vi "LF Read File (STR)__ogtk.vi"(4 "type":string, 5 "convert eol (F)":bool, 6 "bytes to read":i32, 7 "line mode (F)":bool, 8 "error in (no error)":errorcluster, 9 "offset in (0)":dbl, 10 "pos mode (current)":enum16{"start", "end", "current"}(ring)=enum."current", 11 "refnum":refnum<file>) -> (0 "error out":errorcluster, 1 "offset out":dbl, 2 "String":string, 3 "refnum out":refnum<file>)   [LabVIEW 2018]
doc: "Reads a string using a double precision number as offset to work for files larger than 2GB."
uses:
  kernel32.dll
panel:
  # "not implemented"
  # "max offset is limited to about\n2^51 (1 000 000 000 000 000)  bytes\nto maintain full resolution of 1 bytes"
  # "LF Read File (STR).vi\n\nPlease visit http://www.OpenG.org to learn about the\nOpen Source LabVIEW software movement.\n\nNOTICE -- YOU MUST LEAVE THIS NOTICE IN PLACE.  PER THE TERMS OF THE LICENSE BELOW, YOU MAY SUBLICENSE THIS SOFTWARE \nIN ANY WAY THAT DOES NOT CONFLICT WITH THIS LICENSE.\n\n### BSD License (http://www.opensource.org/licenses/bsd-license.php) Begin ###\n\nCopyright (c) 2003, Rolf Kalbermatter <rolf.kalbermatter@citeng.com>\n\nAll rights reserved.\n\nRedistribution and use in source and binary forms, with or without modification, are permitted provided that the following conditions are met:\n\n    * Redistributions of source code must retain the above copyright notice, this list of conditions and the following disclaimer.\n    * Redistributions in binary form must reproduce the above copyright notice, this list of conditions and the following disclaimer in the \n       documentation and/or other materials provided with the distribution.\n    * Neither the name of SciWare, James Kring, Inc., nor the names of its contributors may be used to endorse or promote products derived \n       from this software without specific prior written permission.\n\nTHIS SOFTWARE IS PROVIDED BY THE COPYRIGHT HOLDERS AND CONTRIBUTORS \"AS IS\" AND ANY EXPRESS OR IMPLIED WARRANTIES, \nINCLUDING, BUT NOT LIMITED TO, THE IMPLIED WARRANTIES OF MERCHANTABILITY AND FITNESS FOR A PARTICULAR PURPOSE ARE \nDISCLAIMED. IN NO EVENT SHALL THE COPYRIGHT OWNER OR CONTRIBUTORS BE LIABLE FOR ANY DIRECT, INDIRECT, INCIDENTAL,\n SPECIAL, EXEMPLARY, OR CONSEQUENTIAL DAMAGES (INCLUDING, BUT NOT LIMITED TO, PROCUREMENT OF SUBSTITUTE GOODS OR \nSERVICES; LOSS OF USE, DATA, OR PROFITS; OR BUSINESS INTERRUPTION) HOWEVER CAUSED AND ON ANY THEORY OF LIABILITY, \nWHETHER IN CONTRACT, STRICT LIABILITY, OR TORT (INCLUDING NEGLIGENCE OR OTHERWISE) ARISING IN ANY WAY OUT OF THE USE \nOF THIS SOFTWARE, EVEN IF ADVISED OF THE POSSIBILITY OF SUCH DAMAGE.\n\n### BSD License End ###"
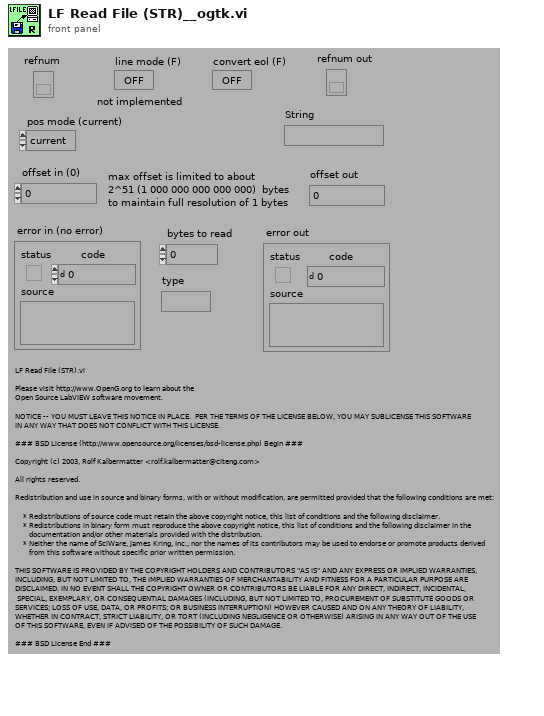
[diagram p1: front panel]
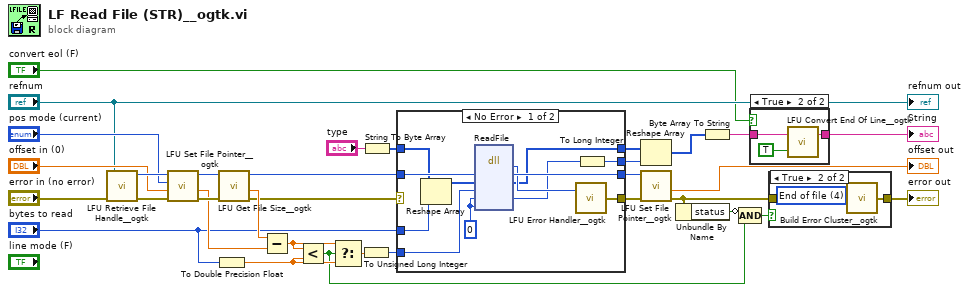
[diagram p0: block diagram]
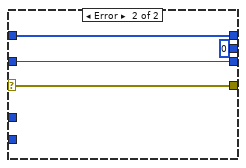
[diagram p4: hidden frame]
diagram:
  n1 = call <userlib>:"LFU Retrieve File Handle__ogtk.vi"("error in (no error)"="error in (no error)", "file refnum"="refnum") -> ("error out"=w31:errorcluster, "handle out"=w32:u32)  [unwired: 4 in]
  n2 = call <userlib>:"LFU Set File Pointer__ogtk.vi"("error in (no error)"=w31, "offset in (0)"="offset in (0)", "pos mode (current)"="pos mode (current)", "handle"=w32) -> ("error out"=w27:errorcluster, "offset out"=w24:dbl, "handle out"=w26:u32)  [unwired: 1 in]
  n3 = To Double Precision Float(number="bytes to read") -> (double precision float=w22:dbl)
  n4 = call <userlib>:"LFU Get File Size__ogtk.vi"("error in (no error)"=w27, "handle"=w26) -> ("error out"=w16:errorcluster, "file size"=w23:dbl, "handle out"=w13:u32)  [unwired: 3 in]
  n5 = Subtract(x=w23, y=w24) -> (x-y=w21:dbl)
  n6 = Less?(x=w21, y=w22) -> (x < y?=w18:bool)
  n7 = Select(t=w21, s=w18, f=w22) -> (s? t:f=w20:dbl)
  n8 = To Unsigned Long Integer(number=w20) -> (unsigned 32bit integer=w14:u32)
  n9 = String To Byte Array(string="type") -> (unsigned byte array=w12:u8[])
  n10 = case shown="No Error" w16 {
    selector: w16 -> [_ w48]
    tunnel: [w45 w49] -> w8
    tunnel: w13 -> [w44 w49]
    tunnel: [w43 w48] -> w4
    tunnel: w14 -> [w41 _]
    tunnel: w12 -> [w39 w47]
    tunnel: "bytes to read" -> [w38 _]
    tunnel: [w36 w47] -> w10
    tunnel: [w35 0 ("bytesRead")] -> w9
    frame No Error {
      w37 = u32 0 ("overlapped")
      n11 = Reshape Array(w39, w38) -> (w40:u8[])
      n12 = dll-call lib="kernel32.dll" fn="ReadFile"("handle"=w44, "buffer"=w40, "bytesToRead"=w41, "bytesRead"=w37, "overlapped"=w37) -> (w42:u32, "handle"=w45:u32, "buffer"=w36:u8[], "bytesRead"=w34:u32)  [unwired: 5 in, 2 out]
      n13 = call <userlib>:"LFU Error Handler__ogtk.vi"("retval"=w42) -> ("error out"=w43:errorcluster)  [unwired: 1 in]
      n14 = To Long Integer(number=w34) -> (32bit integer=w35:i32)
    }
    frame Error {
      (unwired) u32 0 ("bytesRead")
    }
  }
  n15 = Reshape Array(w10, w9) -> (w7:u8[])
  n16 = call <userlib>:"LFU Set File Pointer__ogtk.vi"("error in (no error)"=w4, "handle"=w8) -> ("error out"=w6:errorcluster, "offset out"=→"offset out":dbl)  [unwired: 3 in, 1 out]
  n17 = Unbundle By Name(w6) -> ("status"=w19:bool)
  n18 = Byte Array To String(unsigned byte array=w7) -> (string=w2:string)
  n19 = Compound Arithmetic op=AND(invert w19, w18) -> (w5:bool)
  n20 = case shown="True" "convert eol (F)" {
    tunnel: w2 -> [w50 w53]
    tunnel: [w50 w52] -> w1
    frame False {
    }
    frame True {
      n21 = call <userlib>:"LFU Convert End Of Line__ogtk.vi"("convert to LV"=TRUE, "input"=w53) -> ("output"=w52:string)  [unwired: 1 in]
    }
  }
  "String" <- w1
  n22 = case shown="True" w5 {
    tunnel: w6 -> [w54 _]
    tunnel: [w54 w56] -> w17
    frame False {
    }
    frame True {
      w55 = 4 items=["No error", "Argument error", "Memory is full", "Out of zone", "End of file", "File already open", "Generic file I/O error", "File not found", "File permission error", "Disk is full", "Duplicate path", "Too many files open", "System feature not enabled", "Resource file not found", "Cannot add resource", "Resource not found", "Image not found", "Image memory error", "Pen does not exist", "Config type invalid", "Config token not found", "Config parse error", "Config memory error", "Bad external code format", "Bad external code offset", "External code not present", "Null window", "Destroy window error", "Null menu", "Print aborted", "Bad print record", "Print driver error", "Windows error during printing", "Memory error during printing", "Print dialog error", "Generic print error", "Invalid device refnum", "Device not found", "Device parameter error", "Device unit error", "Cannot open device", "Device call aborted", "Generic error", "Cancelled by user", "Object ID too low", "Object ID too high", "Object not in heap", "Unknown heap", "Unknown object (invalid DefProc)", "Unknown object (DefProc not in table)", "Message out of range", "Invalid (null) method", "Unknown message", "Manager call not supported", "Bad address", "Network operation in progress", "Network operation timed out", "Connection is busy", "Network attribute not supported", "Network error", "Address in use", "System out of memory", "Connection aborted", "Connection refused", "Not connected", "Already connected", "Connection closed", "Initialization error (interapplication manager)", "Bad occurrence", "Wait on unbound occurrence handler", "Occurrence queue overflow", "Datalog type conflict", "Unused", "Unrecognized type (interapplication manager)", "Memory corrupt", "Failed to make temporary DLL", "Old CIN version", "Drag socket not found", "Failed to load drop-object", "Failed to register OLE object", "Failed to release OLE object", "Format specifier type mismatch", "Unknown format specifier", "Too few format specifiers", "Too many format specifiers", "Scan failed", "Newer CIN version", "Error converting to variant", "Runtime menu error", "Password tampered", "Variant attribute not found", "Incompatible variant data type", "Event data is not available", "Event Store is not present", "Occurrence is not found", "Event Queue is not created", "Event info is not available", "Refnum passed is NULL", "Error retrieving Class GUID", "Error retrieving CoClass GUID", "Error retrieving TypeLib GUID.", "Bad built application magic bytes.", "Specific driver is different from the specific driver associated with the Logical Name.", "There is no session opened to the class driver.", "Max Error", "MAX - Error with config objects", "MAX - Error loading configuration", "MAX - Group not supported"]
      n23 = call <userlib>:"Build Error Cluster__ogtk.vi"("code"=w55) -> ("error out"=w56:errorcluster)  [unwired: 1 in]
    }
  }
  "error out" <- w17
  "refnum out" <- "refnum"
